vi "log_file.write.vi"(10 "trace string":string) -> ()   [LabVIEW 2020, in "Nominal Client.lvclass"]
uses:
  Nominal Client.lvclass
  <vilib>/Utility/sysdir.llb/System Directory Type.ctl
  Nominal Client.lvclass/Nominal Client.ctl
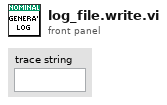
[diagram p1: front panel]
types:
  T1 = enum16{"open", "replace", "create", "open or create", "replace or create", "replace or create with confirmation"}
  T2 = typedef "System Directory Type.ctl" = i32
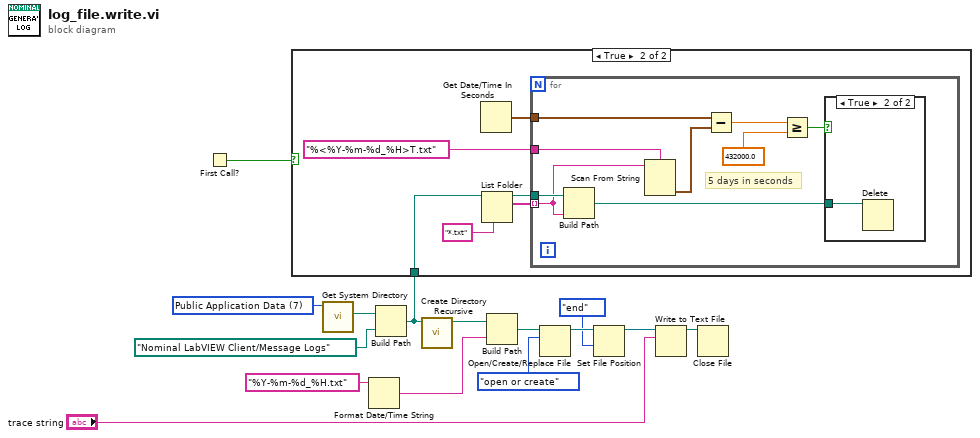
[diagram p0: block diagram]
diagram:
  w15 = T2 7 items=["User Home"=0, "User Desktop"=1, "User Documents"=2, "User Application Data"=3, "User Preferences"=4, "User Temporary"=5, "Public Documents"=6, "Public Application Data"=7, "Public Preferences"=8, "Public Cache"=13, "System Core Libraries"=9, "System Installed Libraries"=10, "Application Files"=11, "Boot Volume Root"=12] ("system directory type")
  n1 = First Call?() -> (First Call?: T/F=w1:bool)
  n2 = call <vilib>:"Get System Directory.vi"("system directory type"=w15) -> ("system directory"=w14:path)  [unwired: 10 in]
  n3 = Format Date/Time String(time format string (%c)="%Y-%m-%d_%H.txt") -> (date/time string=w7:string)  [unwired: 2 in]
  n4 = Build Path(base path=w14, name or relative path=path "Nominal LabVIEW Client/Message Logs") -> (appended path=w2:path)
  n5 = case shown="True" w1 {
    tunnel: w2 -> [_ w21]
    frame False {
    }
    frame True {
      n6 = Get Date/Time In Seconds() -> (seconds since 1Jan1904=w16:timestamp)
      n7 = List Folder(path=w21, pattern="*.txt") -> (path out=w20:path, filenames=w19:string[])  [unwired: 2 in, 2 out]
      n8 = for {
        tunnel: w20 -> [w30]
        tunnel: w19 -> [w28] mode=indexing
        tunnel: "%<%Y-%m-%d_%H>T.txt" ("time format string (%c)") -> [w29]
        tunnel: w16 -> [w27]
        # "5 days in seconds"
        n9 = Build Path(base path=w30, name or relative path=w28) -> (appended path=w22:path)
        n10 = Scan From String(format string=w29, input string=w28) -> (output 1=w26:timestamp)  [unwired: 3 in, 3 out]
        n11 = Subtract(x=w27, y=w26) -> (x-y=w25:dbl)
        n12 = Greater Or Equal?(x=w25, y=432000.0) -> (x >= y?=w23:bool)
        n13 = case shown="True" w23 {
          tunnel: w22 -> [_ w31]
          frame False {
          }
          frame True {
            n14 = Delete(path (use dialog)=w31) -> ()  [unwired: 4 in, 3 out]
          }
        }
      }
    }
  }
  n15 = call <vilib>:"Create Directory Recursive.vi"("directory"=w2) -> ("directory copy"=w6:path)  [unwired: 4 in, 2 out]
  n16 = Build Path(base path=w6, name or relative path=w7) -> (appended path=w8:path)
  n17 = Open/Create/Replace File(file path (use dialog)=w8, operation (0:open)=T1."open or create") -> (refnum out=w5:refnum<file>)  [unwired: 4 in, 2 out]
  n18 = Set File Position(refnum=w5, from (0:start)=enum16{"start", "end", "current"}."end") -> (refnum out=w4:refnum<file>)  [unwired: 2 in, 1 out]
  n19 = Write to Text File(file (use dialog)=w4, text="trace string") -> (refnum out=w11:refnum<file>)  [unwired: 2 in, 2 out]
  n20 = Close File(refnum=w11) -> ()  [unwired: 1 in, 2 out]
